vi "Get_Set_Device.vi"(6 "Get/Set":T4, 7 "Element":T3=enum."Master?", 8 "Status/Errors in":refnum<vi>, 9 "Device in":refnum<vi>, 10 "Value in":variant) -> (0 "Status/Errors out":refnum<vi>, 1 "Device out":refnum<vi>, 2 "Value out":variant, 3 "Device":T2, 4 "Connected?":bool, 5 "Master?":T1)   [LabVIEW 2010]
uses:
  Controls/Get_Set_Device_Options.ctl
  Controls/Device_Elements.ctl
  Controls/Device.ctl
  Controls/Master.ctl
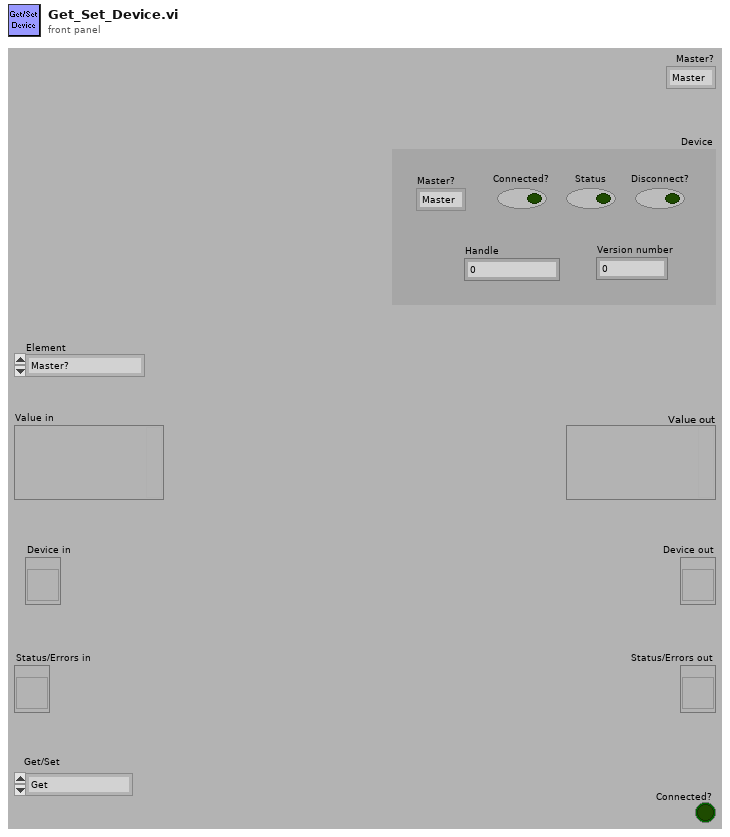
[diagram p1: front panel]
types:
  T1 = typedef "Master.ctl" = enum16{"Master", "Slave", "General"}
  T2 = typedef "Device.ctl" = cluster{"Master?":T1, "Connected?":bool, "Status":bool, "Disconnect?":bool, "Handle":u32, "Version number":u32}
  T3 = typedef "Device_Elements.ctl" = enum16{"Default", "Master?", "Connected?", "Status", "Disconnect?", "Handle", "Version number"}
  T4 = typedef "Get_Set_Device_Options.ctl" = enum16{"Get", "Get cluster", "Set"}
  T5 = cluster{"Master?":T1, "Connected?":bool, "Status":bool, "Disconnect?":bool, "Handle":u32, "Version number":u32}
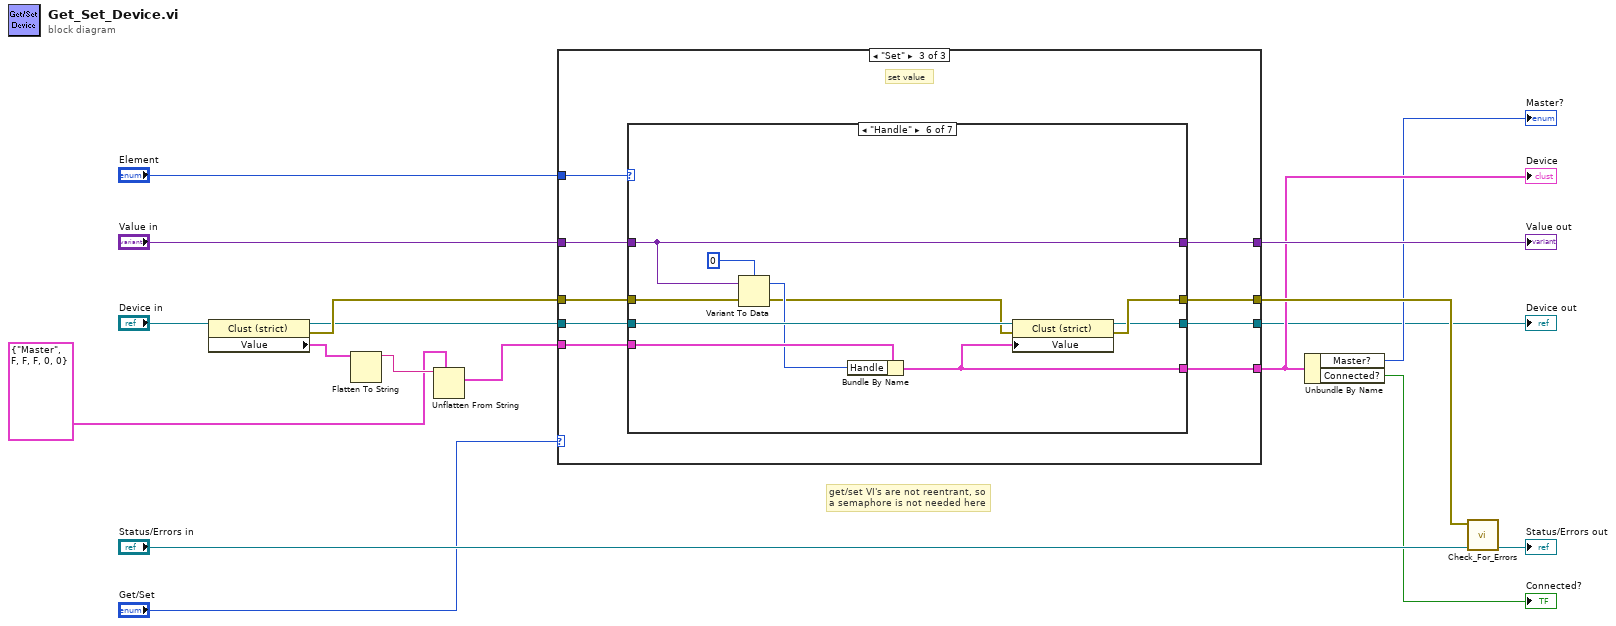
[diagram p0: block diagram]
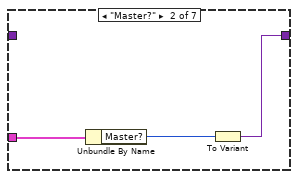
[diagram p3: hidden frame]
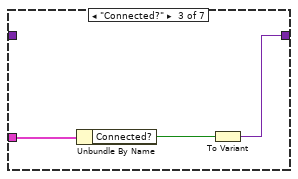
[diagram p4: hidden frame]
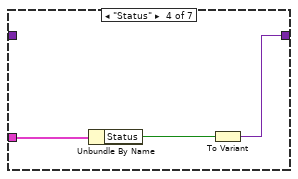
[diagram p5: hidden frame]
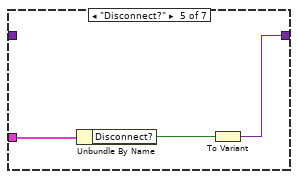
[diagram p6: hidden frame]
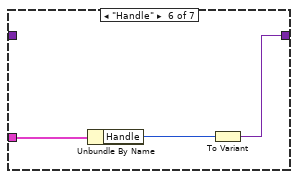
[diagram p7: hidden frame]
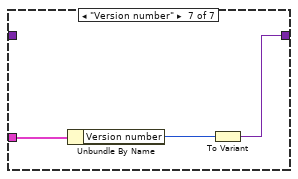
[diagram p8: hidden frame]
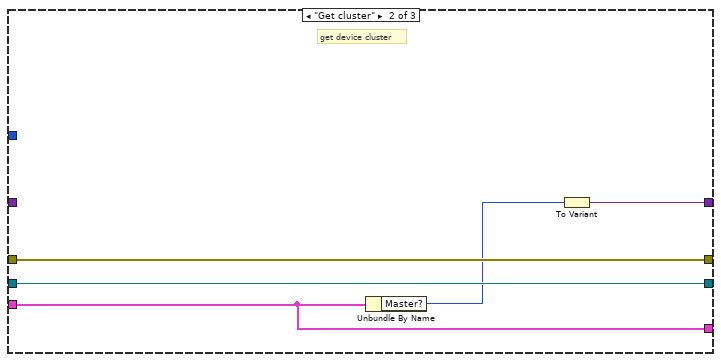
[diagram p9: hidden frame]
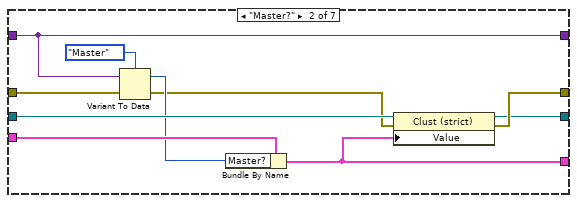
[diagram p11: hidden frame]
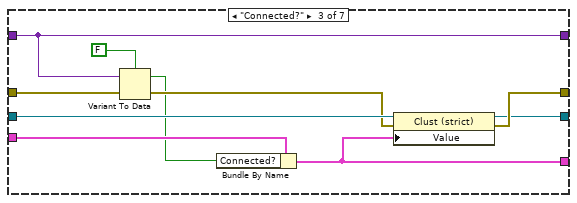
[diagram p12: hidden frame]
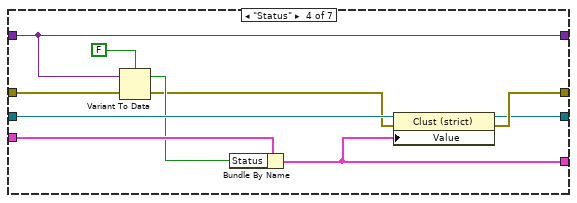
[diagram p13: hidden frame]
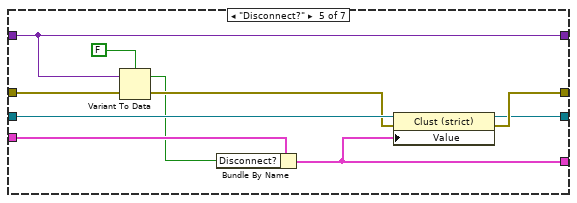
[diagram p14: hidden frame]
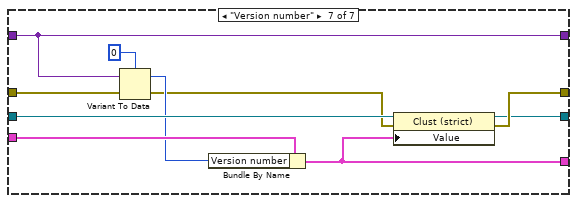
[diagram p15: hidden frame]
diagram:
  # "get/set VI's are not reentrant, so\na semaphore is not needed here"
  n1 = property class="Clust (strict)"(reference="Device in") -> (reference out=w1:refnum<vi>, error out=w11:errorcluster, "Value"=w16:T5)  [unwired: 1 in]
  n2 = Flatten To String(anything=w16) -> (data string=w15:string)  [unwired: 1 in, 4 out]
  n3 = Unflatten From String(type=T2 {"Master?"=enum."Master", "Connected?"=FALSE, "Status"=FALSE, "Disconnect?"=FALSE, "Handle"=0, "Version number"=0} ("Device"), binary string=w15) -> (value=w7:T2)  [unwired: 1 in, 4 out]
  n4 = case shown="\"Set\"" "Get/Set" {
    tunnel: "Element" -> [w24 _ w57]
    tunnel: w7 -> [w19 w44 w50]
    tunnel: "Value in" -> [w20 _ w56]
    tunnel: w11 -> [w23 w47 w55]
    tunnel: w1 -> [w21 w48 w54]
    tunnel: [w21 w48 w53] -> w3
    tunnel: [w23 w47 w52] -> w9
    tunnel: [w22 w46 w51] -> w12
    tunnel: [w19 w44 w49] -> w6
    frame "Get" {
      # "get value"
      n5 = case shown="Default" w24 {
        tunnel: w19 -> [_ w28 w31 w34 w37 w40 w43]
        tunnel: [w25 w26 w29 w32 w35 w38 w41] -> w22
        tunnel: w20 -> [w25 _ _ _ _ _ _]
        frame Default {
        }
        frame "Master?" {
          n6 = Unbundle By Name(w28) -> ("Master?"=w27:T1)
          n7 = To Variant(anything=w27) -> (Variant=w26:variant)
        }
        frame "Connected?" {
          n8 = Unbundle By Name(w31) -> ("Connected?"=w30:bool)
          n9 = To Variant(anything=w30) -> (Variant=w29:variant)
        }
        frame "Status" {
          n10 = Unbundle By Name(w34) -> ("Status"=w33:bool)
          n11 = To Variant(anything=w33) -> (Variant=w32:variant)
        }
        frame "Disconnect?" {
          n12 = Unbundle By Name(w37) -> ("Disconnect?"=w36:bool)
          n13 = To Variant(anything=w36) -> (Variant=w35:variant)
        }
        frame "Handle" {
          n14 = Unbundle By Name(w40) -> ("Handle"=w39:u32)
          n15 = To Variant(anything=w39) -> (Variant=w38:variant)
        }
        frame "Version number" {
          n16 = Unbundle By Name(w43) -> ("Version number"=w42:u32)
          n17 = To Variant(anything=w42) -> (Variant=w41:variant)
        }
      }
    }
    frame "Get cluster" {
      # "get device cluster"
      n18 = Unbundle By Name(w44) -> ("Master?"=w45:T1)
      n19 = To Variant(anything=w45) -> (Variant=w46:variant)
    }
    frame "Set" {
      # "set value"
      n20 = case shown="\"Handle\"" w57 {
        tunnel: w50 -> [w58 w71 w81 w91 w101 w111 w121]
        tunnel: w56 -> [w59 w64 w74 w83 w94 w104 w114]
        tunnel: w55 -> [w60 w70 w80 w90 w100 w110 w120]
        tunnel: w54 -> [w61 w69 w79 w89 w99 w109 w119]
        tunnel: [w61 w65 w75 w84 w95 w105 w115] -> w53
        tunnel: [w60 w66 w76 w85 w96 w106 w116] -> w52
        tunnel: [w59 w64 w74 w83 w94 w104 w114] -> w51
        tunnel: [w58 w62 w72 w82 w92 w102 w112] -> w49
        frame Default {
        }
        frame "Master?" {
          n21 = Variant To Data(error in=w70, Variant=w64, type=Master."Master" ("Master?")) -> (error out=w67:errorcluster, data=w68:T1)
          n22 = Bundle By Name(cluster=w71, "Master?"=w68) -> (w62:T2)
          n23 = property class="Clust (strict)"(reference=w69, error in=w67, "Value"=w62) -> (reference out=w65:refnum<vi>, error out=w66:errorcluster)
        }
        frame "Connected?" {
          n24 = Variant To Data(error in=w80, Variant=w74, type=FALSE) -> (error out=w78:errorcluster, data=w73:bool)
          n25 = Bundle By Name(cluster=w81, "Connected?"=w73) -> (w72:T2)
          n26 = property class="Clust (strict)"(reference=w79, error in=w78, "Value"=w72) -> (reference out=w75:refnum<vi>, error out=w76:errorcluster)
        }
        frame "Status" {
          n27 = Variant To Data(error in=w90, Variant=w83, type=FALSE) -> (error out=w87:errorcluster, data=w88:bool)
          n28 = Bundle By Name(cluster=w91, "Status"=w88) -> (w82:T2)
          n29 = property class="Clust (strict)"(reference=w89, error in=w87, "Value"=w82) -> (reference out=w84:refnum<vi>, error out=w85:errorcluster)
        }
        frame "Disconnect?" {
          n30 = Variant To Data(error in=w100, Variant=w94, type=FALSE) -> (error out=w98:errorcluster, data=w93:bool)
          n31 = Bundle By Name(cluster=w101, "Disconnect?"=w93) -> (w92:T2)
          n32 = property class="Clust (strict)"(reference=w99, error in=w98, "Value"=w92) -> (reference out=w95:refnum<vi>, error out=w96:errorcluster)
        }
        frame "Handle" {
          n33 = Variant To Data(error in=w110, Variant=w104, type=u32 0) -> (error out=w107:errorcluster, data=w108:u32)
          n34 = Bundle By Name(cluster=w111, "Handle"=w108) -> (w102:T2)
          n35 = property class="Clust (strict)"(reference=w109, error in=w107, "Value"=w102) -> (reference out=w105:refnum<vi>, error out=w106:errorcluster)
        }
        frame "Version number" {
          n36 = Variant To Data(error in=w120, Variant=w114, type=0 ("Device id")) -> (error out=w117:errorcluster, data=w118:i32)
          n37 = Bundle By Name(cluster=w121, "Version number"=w118) -> (w112:T2)
          n38 = property class="Clust (strict)"(reference=w119, error in=w117, "Value"=w112) -> (reference out=w115:refnum<vi>, error out=w116:errorcluster)
        }
      }
    }
  }
  "Value out" <- w12
  "Device" <- w6
  "Device out" <- w3
  n39 = Unbundle By Name(w6) -> ("Master?"=→"Master?":T1, "Connected?"=→"Connected?":bool)
  n40 = call "Check_For_Errors.vi"("Status/Errors in"="Status/Errors in", "error in"=w9) -> ("Status/Errors out"=→"Status/Errors out":refnum<vi>)  [unwired: 9 out]
